vi "Code 0.0.5.vi"(8 "error in (no error)":errorcluster, 9 "Drv":u8(ring) items=["Drv 1", "Drv 2"], 10 "Port":u16=8030) -> (0 "error out":errorcluster)   [LabVIEW 2017]
panel:
  out "DataOut1":string
  out "DataOut2":string
  out "2":i32[][](array[numeric])
  out "1":i32[](array[numeric])
  in  "StopS.M. 2":bool
  in  "StopS.M.":bool
  in  "CatchNetworkFlag":bool
  in  "stop Listen":bool
  in  "status":bool
  out "conn ID":refnum<k5>
  out "Error List":string
  in  "Next Button":bool
  in  "File Path Control":path
  out "Status":bool
  out "CheckSum":bool[][](array[boolean])
  out "CheckSum DataB":u16 format="%.0x"
  out "CheckSum Data":u16 format="%.0x"
  out "Writting Data":bool
  out "Send Header":bool
  out "sumHeader":u16 format="%.0x"
  # "Ver 0.0.7"
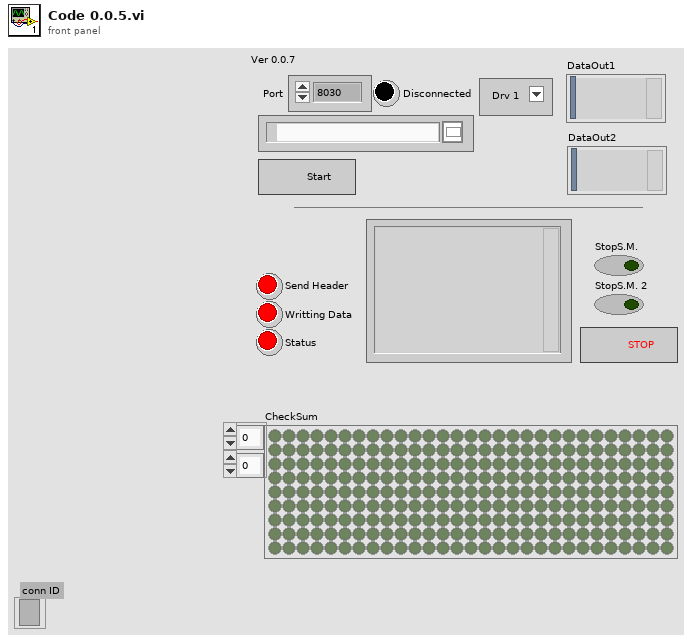
[diagram p1: front panel]
types:
  T1 = enum16{"open", "replace", "create", "open or create", "replace or create", "replace or create with confirmation"}
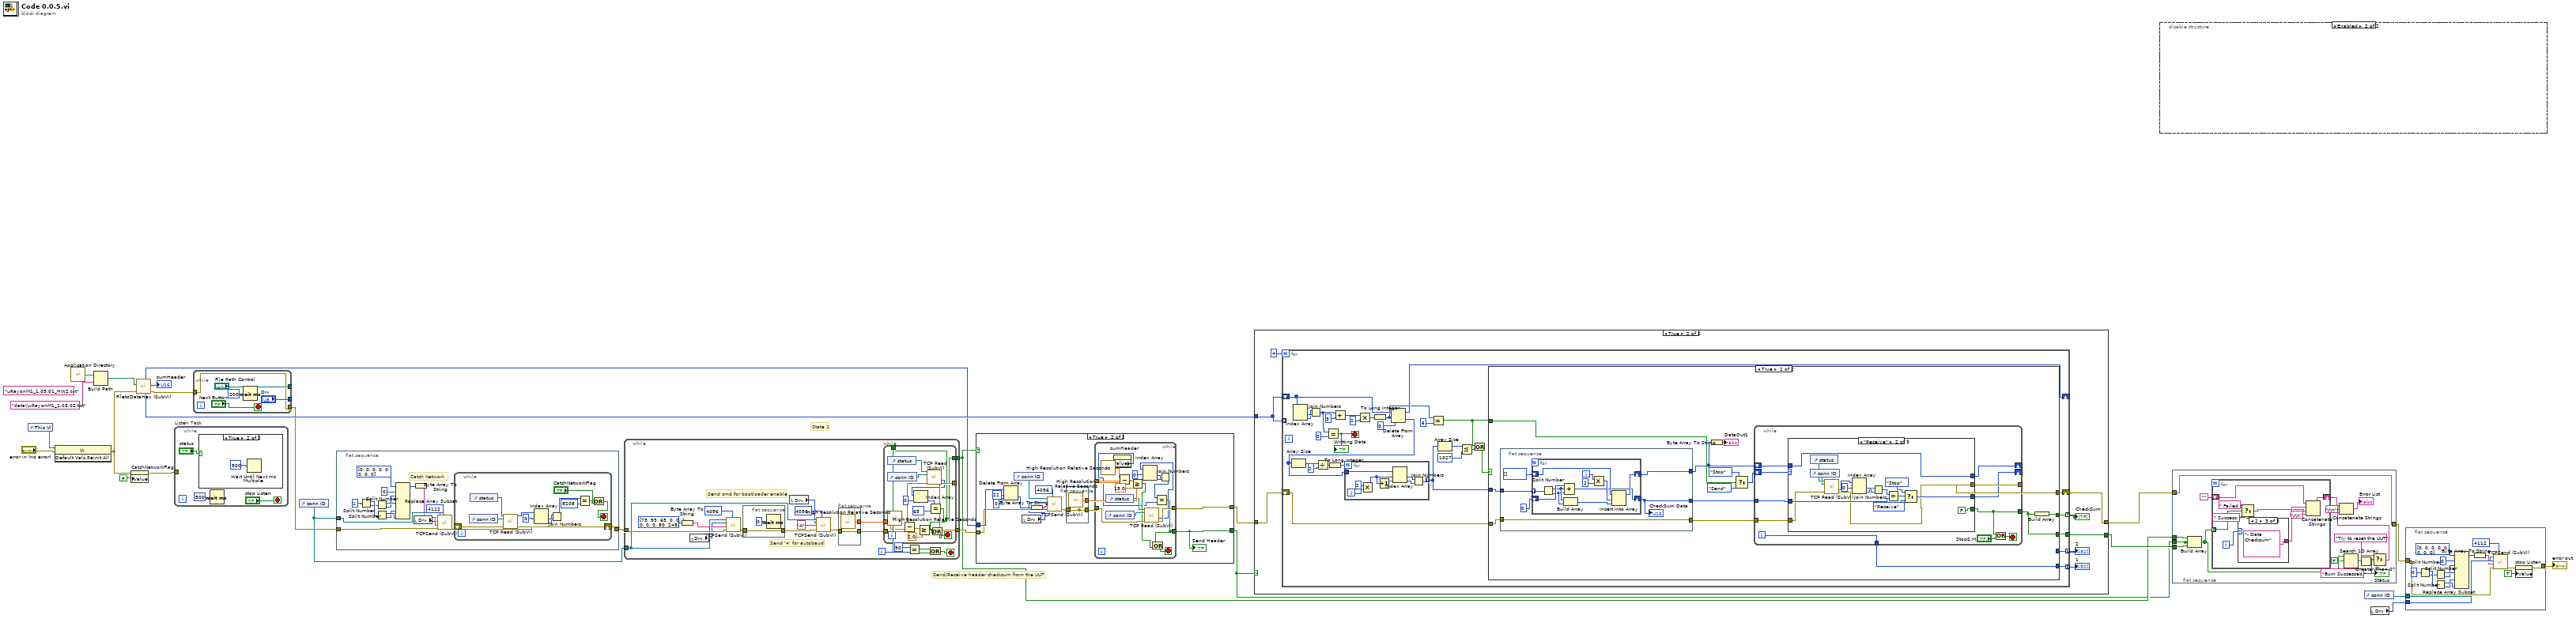
[diagram p0: block diagram]
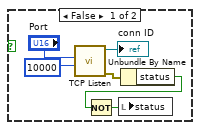
[diagram p2: hidden frame]
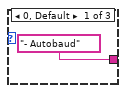
[diagram p3: hidden frame]
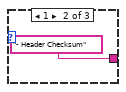
[diagram p4: hidden frame]
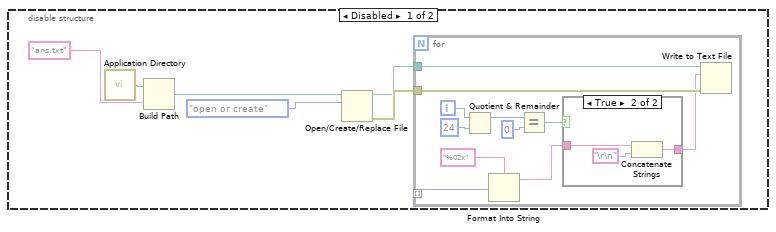
[diagram p5: hidden frame]
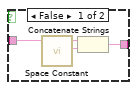
[diagram p6: hidden frame]
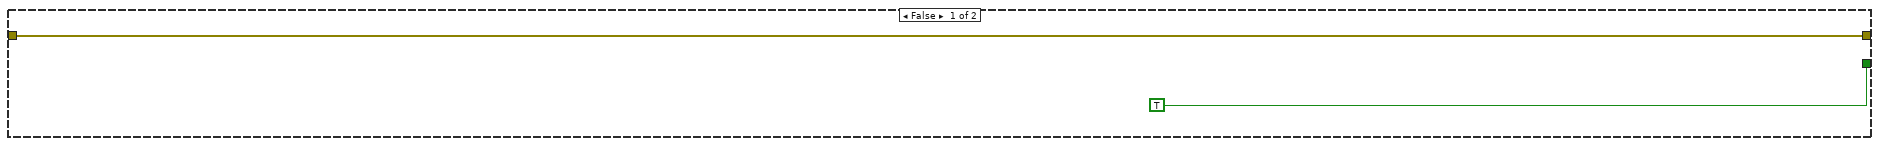
[diagram p7: hidden frame]
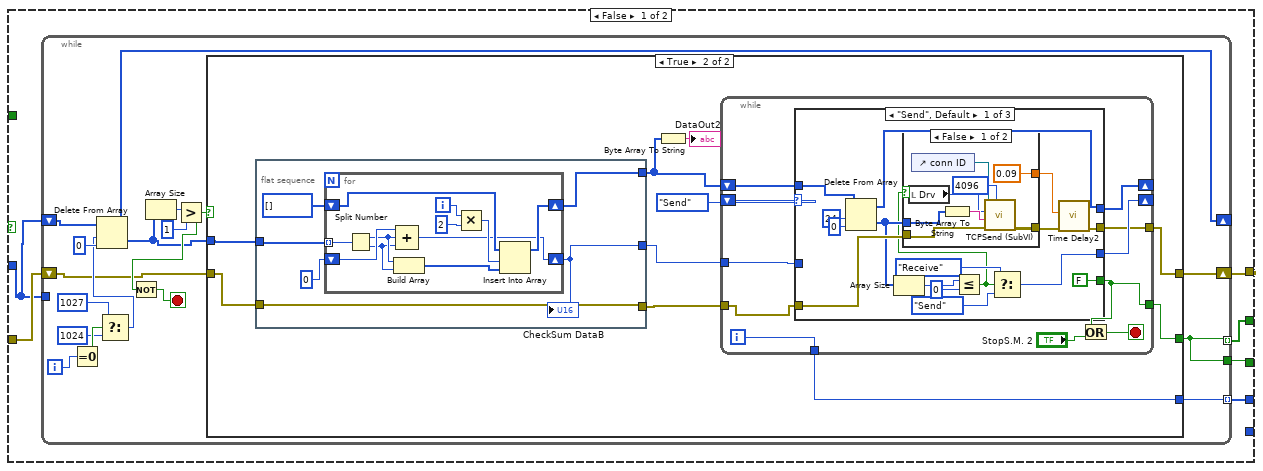
[diagram p8: hidden frame]
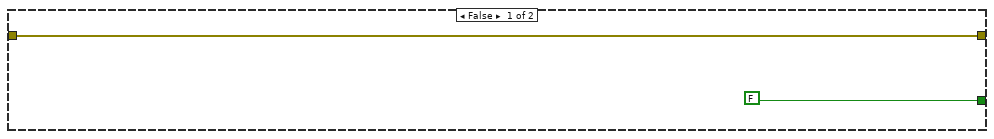
[diagram p9: hidden frame]
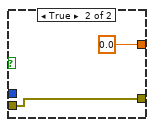
[diagram p10: hidden frame]
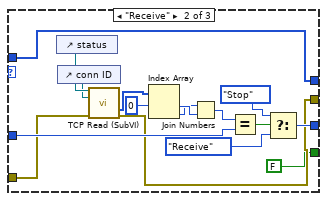
[diagram p11: hidden frame]
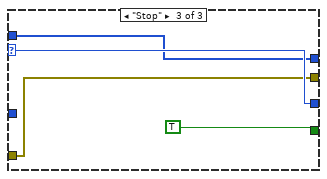
[diagram p12: hidden frame]
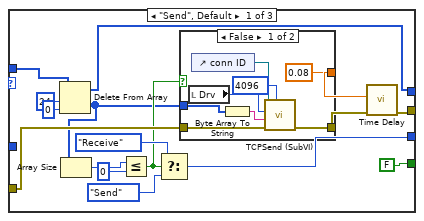
[diagram p13: hidden frame]
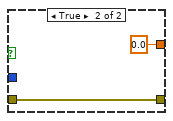
[diagram p14: hidden frame]
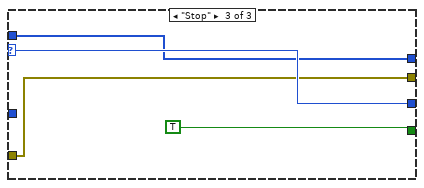
[diagram p15: hidden frame]
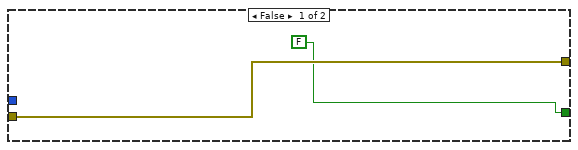
[diagram p16: hidden frame]
diagram:
  (unwired) "uRayonM1_1.05.01_HW2.txt" ("name or relative path")
  # "State 1"
  # "Send/Receive header checksum from the UUT"
  n1 = control-ref of="This VI"() -> (w24:refnum<vi>)
  n2 = invoke class="VI" method="Default Vals.Reinit All"(reference=w24, error in="error in (no error)") -> (error out=w4:errorcluster)  [unwired: 1 in, 2 out]
  n3 = call <vilib>:"Application Directory.vi"() -> ("Application Directory"=w8:path)
  n4 = Build Path(base path=w8, name or relative path="data\\uRayonM1_1.03.02.txt") -> (appended path=w7:path)
  n5 = property on="CatchNetworkFlag" class="Bool (strict)"(error in=w4, "Value"=FALSE ("stop")) -> (error out=w17:errorcluster)  [unwired: 1 in, 1 out]
  n6 = call "FiletoDataHex (SubVI).vi"("error constant"=w4, "file path (use dialog)"=w7) -> ("error constant 2"=w6:errorcluster, "Array 2"=w25:u8[], "Array"=w20:u8[], "sumHeader"=→"sumHeader":u16)  [unwired: 3 in, 3 out]
  n7 = while "Listen Task" {
    tunnel: w17 -> [_]
    stop <- "stop Listen" stop-if-true
    n8 = case shown="True" "status" {
      frame False {
        n9 = call <vilib>:"TCP Listen.vi"("timeout ms (wait forever: -1)"=10000, "port"="Port") -> ("error out"=w32:errorcluster, "connection ID"=→"conn ID":refnum<k5>)  [unwired: 5 in, 3 out]
        n10 = Unbundle By Name(w32) -> ("status"=w29:bool)
        n11 = Not(x=w29) -> (.not. x?=w30:bool)
        n12 = local write "status"(w30) -> ()
      }
      frame True {
        n13 = Wait Until Next ms Multiple(millisecond multiple=u32 500) -> ()  [unwired: 1 out]
      }
    }
    n14 = Wait (ms)(milliseconds to wait=u32 500) -> ()  [unwired: 1 out]
  }
  n15 = while {
    tunnel: ["File Path Control"] -> _
    tunnel: w6 -> [w36]
    tunnel: ["Drv"] -> _
    tunnel: [w36] -> w11
    stop <- "Next Button" stop-if-true
    n16 = Wait (ms)(milliseconds to wait=u32 200) -> ()  [unwired: 1 out]
  }
  n17 = control-ref of="conn ID"() -> (w13:refnum<vi>)
  n18 = flat-sequence {
    tunnel: w11 -> [w56]
    tunnel: w13 -> [w55]
    tunnel: [w43] -> w22
    frame #0 {
      # "Catch Network"
      n19 = Split Number(x=u32 1) -> (hi(x)=w53:u16, lo(x)=w52:u16)
      n20 = Split Number(x=w52) -> (hi(x)=w47:u8, lo(x)=w46:u8)
      n21 = Split Number(x=w53) -> (hi(x)=w45:u8, lo(x)=w44:u8)
      n22 = Replace Array Subset(array=u8[] [0, 0, 0, 0, 0, 0, 0, 0] ("unsigned byte array"), new element #1=w46, index #1=0 ("index"), new element #2=w47, new element #3=w44, new element #4=w45) -> (w48:u8[])  [unwired: 3 in]
      n23 = Byte Array To String(unsigned byte array=w48) -> (string=w54:string)
      n24 = local read "Drv"() -> (w41:u8)
      n25 = call "TCPSend (SubVI).vi"("Opcode"=u32 4112, "error in"=w56, "string"=w54, "Drv"=w41, "RefNum in"=w55) -> ("error out"=w42:errorcluster)  [unwired: 6 in]
      n26 = while {
        shift-right: [w69] -> w43
        shift-left: w42 -> [w70]
        stop <- w64 stop-if-true
        n27 = control-ref of="conn ID"() -> (w62:refnum<vi>)
        n28 = control-ref of="status"() -> (w63:refnum<vi>)
        n29 = call "TCP Read (SubVI).vi"("Status in"=w63, "TCP in"=w62, "error in (no error)"=w70) -> ("Rx data tmp"=w61:u8[], "error out"=w69:errorcluster)  [unwired: 2 in, 9 out]
        n30 = Index Array(array=w61, index #1=0 ("index")) -> (element #1=w60:u8, element #2=w59:u8)  [unwired: 1 in]
        n31 = Join Numbers(hi=w59, lo=w60) -> ((hi.lo)=w68:u16)
        n32 = Equal?(x=w68, y=u16 8208) -> (x = y?=w66:bool)
        n33 = Or(x="CatchNetworkFlag", y=w66) -> (x .or. y?=w64:bool)
      }
    }
  }
  n34 = while {
    tunnel: w22 -> [w84]
    tunnel: [w81] -> w16
    tunnel: w13 -> [w91]
    tunnel: [w80] -> w5
    i -> [w88]
    stop <- w90 stop-if-true
    # "Send 'A' for autobaud"
    # "Send cmd for bootloader enable"
    n35 = Byte Array To String(unsigned byte array=u8[] [73, 93, 65, 0, 0, 1, 0, 0, 0, 80, 248] ("output array")) -> (string=w76:string)
    n36 = local read "Drv"() -> (w71:u8)
    n37 = call "TCPSend (SubVI).vi"("Opcode"=u32 4096, "error in"=w84, "string"=w76, "Drv"=w71, "RefNum in"=w91) -> ("error out"=w78:errorcluster)  [unwired: 6 in]
    n38 = flat-sequence {
      tunnel: w78 -> [w92]
      tunnel: [w92] -> w77
      frame #0 {
        n39 = Wait (ms)(milliseconds to wait=u32 0) -> ()  [unwired: 1 out]
      }
    }
    n40 = local read "Drv"() -> (w72:u8)
    n41 = call "TCPSend (SubVI).vi"("Opcode"=u32 4096, "error in"=w77, "string"="A" ("write buffer"), "Drv"=w72, "RefNum in"=w91) -> ("error out"=w82:errorcluster)  [unwired: 6 in]
    n42 = flat-sequence {
      tunnel: w82 -> [w95]
      tunnel: [w95] -> w86
      tunnel: [w94] -> w85
      frame #0 {
        n43 = call <vilib>:"High Resolution Relative Seconds.vi"() -> ("relative seconds"=w94:dbl)
      }
    }
    n44 = while {
      tunnel: w86 -> [w99]
      tunnel: w85 -> [w105]
      tunnel: [w98] -> w81
      tunnel: [w96] -> w83
      tunnel: [w96] -> w80
      stop <- w97 stop-if-true
      n45 = control-ref of="status"() -> (w109:refnum<vi>)
      n46 = control-ref of="conn ID"() -> (w110:refnum<vi>)
      n47 = call <vilib>:"High Resolution Relative Seconds.vi"() -> ("relative seconds"=w106:dbl)
      n48 = Subtract(x=w106, y=w105) -> (x-y=w104:dbl)
      n49 = Greater Or Equal?(x=w104, y=2.0) -> (x >= y?=w102:bool)
      n50 = call "TCP Read (SubVI).vi"("Status in"=w109, "TCP in"=w110, "error in (no error)"=w99) -> ("Drv Array"=w107:u8[], "error out"=w98:errorcluster)  [unwired: 2 in, 9 out]
      n51 = Index Array(array=w107, index=0) -> (element=w101:u8)
      n52 = Equal?(x=w101, y=u8 65) -> (x = y?=w96:bool)
      n53 = Or(x=w96, y=w102) -> (x .or. y?=w97:bool)
    }
    n54 = Equal?(x=90, y=w88) -> (x = y?=w89:bool)
    n55 = Compound Arithmetic op=OR(w89, w83) -> (w90:bool)
  }
  n56 = case shown="True" w5 {
    tunnel: w16 -> [w112 w124]
    tunnel: [w112 w126] -> w2
    tunnel: w20 -> [_ w125]
    tunnel: [FALSE w114] -> w1
    frame False {
    }
    frame True {
      n57 = Delete From Array(array=w125, length=22, index=0) -> (deleted portion=w120:u8[])  [unwired: 1 out]
      n58 = control-ref of="conn ID"() -> (w117:refnum<vi>)
      n59 = local read "Drv"() -> (w113:u8)
      n60 = Byte Array To String(unsigned byte array=w120) -> (string=w118:string)
      n61 = call "TCPSend (SubVI).vi"("Opcode"=u32 4096, "error in"=w124, "string"=w118, "Drv"=w113, "RefNum in"=w117) -> ("error out"=w123:errorcluster)  [unwired: 6 in]
      n62 = flat-sequence {
        tunnel: w123 -> [w127]
        tunnel: [w127] -> _
        tunnel: [w128] -> w115
        tunnel: [w127] -> w116
        frame #0 {
          n63 = call <vilib>:"High Resolution Relative Seconds.vi"() -> ("relative seconds"=w128:dbl)
        }
      }
      n64 = while {
        tunnel: w116 -> [w139]
        tunnel: [w138] -> w126
        tunnel: w115 -> [w144]
        tunnel: [w129] -> w114
        stop <- w135 stop-if-true
        n65 = call <vilib>:"High Resolution Relative Seconds.vi"() -> ("relative seconds"=w145:dbl)
        n66 = control-ref of="status"() -> (w141:refnum<vi>)
        n67 = control-ref of="conn ID"() -> (w140:refnum<vi>)
        n68 = property on="sumHeader" class="DigNum (strict)"() -> ("Value"=w130:u16)  [unwired: 2 in, 2 out]
        n69 = Subtract(x=w145, y=w144) -> (x-y=w143:dbl)
        n70 = Greater Or Equal?(x=w143, y=15.0) -> (x >= y?=w134:bool)
        n71 = call "TCP Read (SubVI).vi"("Status in"=w141, "TCP in"=w140, "error in (no error)"=w139) -> ("Drv Array"=w136:u8[], "error out"=w138:errorcluster)  [unwired: 2 in, 9 out]
        n72 = Index Array(array=w136, index #1=0 ("index")) -> (element #1=w132:u8, element #2=w133:u8)  [unwired: 1 in]
        n73 = Join Numbers(hi=w133, lo=w132) -> ((hi.lo)=w131:u16)
        n74 = Equal?(x=w131, y=w130) -> (x = y?=w129:bool)
        n75 = Compound Arithmetic op=OR(w129, w134) -> (w135:bool)
      }
      "Send Header" <- w114
    }
  }
  n76 = case shown="True" w1 {
    tunnel: w2 -> [w147 w153]
    tunnel: [w147 w152] -> w19
    tunnel: w25 -> [_ w155]
    tunnel: [TRUE w151] -> w23
    frame False {
    }
    frame True {
      n77 = for {
        N: 4 -> [_]
        shift-right: [w176] -> _
        shift-left: w155 -> [w186]
        tunnel: w155 -> [_] mode=indexing
        tunnel: [w165] -> w154 mode=indexing
        shift-right: [w158] -> w152
        shift-left: w153 -> [w160]
        tunnel: [w159] -> w151
        tunnel: [w157] -> w149 mode=indexing
        tunnel: [w156] -> w148 mode=indexing
        stop <- w179 stop-if-true
        n78 = Index Array(array=w186) -> (element #1=w185:u8, element #2=w184:u8)  [unwired: 2 in]
        n79 = Join Numbers(hi=w184, lo=w185) -> ((hi.lo)=w162:u16)
        n80 = Equal?(x=w162, y=u16 0) -> (x = y?=w179:bool)
        "Writting Data" <- w179
        n81 = Add(x=w162, y=u32 3) -> (x+y=w182:u32)
        n82 = Multiply(x=w182, y=u32 2) -> (x*y=w180:u32)
        n83 = To Long Integer(number=w180) -> (32bit integer=w163:i32)
        n84 = Delete From Array(array=w186, length=w163, index=0) -> (deleted portion=w164:u8[], array with subset deleted=w176:u8[])
        n85 = Array Size(array=w164) -> (size(s)=w173:i32)
        n86 = Divide(x=w173, y=2) -> (x/y=w175:dbl)
        n87 = To Long Integer(number=w175) -> (32bit integer=w172:i32)
        n88 = for {
          N: w172 -> [_]
          tunnel: w164 -> [w388]
          tunnel: [w384] -> w169 mode=indexing
          i -> [w387]
          n89 = Multiply(x=2, y=w387) -> (x*y=w390:i32)
          n90 = Increment(x=w390) -> (x+1=w391:i32)
          n91 = Index Array(array=w388, index #1=w390, index #2=w391) -> (element #1=w386:u8, element #2=w385:u8)
          n92 = Join Numbers(hi=w386, lo=w385) -> ((hi.lo)=w384:u16)
        }
        n93 = Equal?(x=w163, y=6) -> (x = y?=w161:bool)
        n94 = Array Size(array=w169) -> (size(s)=w171:i32)
        n95 = Less Or Equal?(x=w171, y=1027) -> (x <= y?=w167:bool)
        n96 = Or(x=w161, y=w167) -> (x .or. y?=w166:bool)
        n97 = case shown="True" w166 {
          tunnel: w160 -> [w191 w307]
          tunnel: [w192 w304] -> w158
          tunnel: w169 -> [w189 w309]
          tunnel: [w190 w308] -> w165
          tunnel: w161 -> [_ w301]
          tunnel: [w188 w299] -> w159
          tunnel: [_ w298] -> w157
          tunnel: [w187 _] -> w156
          frame False {
            n98 = while {
              tunnel: w189 -> [_]
              tunnel: [w195] -> w190 mode=indexing
              shift-right: [w209] -> w192
              shift-left: w191 -> [w196]
              shift-right: [w202] -> _
              shift-left: w189 -> [w208]
              tunnel: [w195] -> w188
              tunnel: [w194] -> w187 mode=indexing
              i -> [w201]
              stop <- w203 stop-if-true
              n99 = Equal To 0?(x=w201) -> (x = 0?=w200:bool)
              n100 = Select(t=1027 ("length"), s=w200, f=1024 ("length")) -> (s? t:f=w197:i32)
              n101 = Delete From Array(array=w208, length=w197, index=0) -> (deleted portion=w193:u16[], array with subset deleted=w202:u16[])
              n102 = Array Size(array=w193) -> (size(s)=w206:i32)
              n103 = Greater?(x=w206, y=1) -> (0:w204:bool)
              n104 = Not(x=w204) -> (.not. x?=w203:bool)
              n105 = case shown="True" w204 {
                tunnel: [w211 w218] -> w209
                tunnel: w196 -> [w211 w220]
                tunnel: [FALSE w216] -> w195
                tunnel: w193 -> [_ w221]
                tunnel: [_ w214] -> w194
                frame False {
                }
                frame True {
                  n106 = flat-sequence {
                    tunnel: w220 -> [w280]
                    tunnel: [w282] -> w213
                    tunnel: [w279] -> w217
                    tunnel: w221 -> [w281]
                    tunnel: [w280] -> w215
                    frame #0 {
                      n107 = for {
                        tunnel: w281 -> [w295] mode=indexing
                        shift-right: [w290] -> w282
                        shift-left: u8[] [] -> [w289]
                        shift-right: [w287] -> w279
                        shift-left: u16 0 -> [w288]
                        i -> [w294]
                        n108 = Split Number(x=w295) -> (hi(x)=w286:u8, lo(x)=w285:u8)
                        n109 = Build Array(w286, w285) -> (w292:u8[])
                        n110 = Compound Arithmetic op=ADD(w288, w286, w285) -> (w287:u16)
                        n111 = Multiply(x=w294, y=2) -> (x*y=w291:i32)
                        n112 = Insert Into Array(array=w289, index=w291, new element=w292) -> (w290:u8[])
                      }
                      "CheckSum DataB" <- w279
                    }
                  }
                  n113 = Byte Array To String(unsigned byte array=w213) -> (string=→"DataOut2":string)
                  n114 = while {
                    shift-right: [w230] -> _
                    shift-left: enum16{"Stop", "Receive", "Send"}."Send" -> [w232]
                    shift-right: [w228] -> _
                    shift-left: w213 -> [w231]
                    tunnel: w215 -> [w223]
                    tunnel: w217 -> [w229]
                    tunnel: [w222] -> w216
                    tunnel: [w227] -> w218
                    tunnel: [w224] -> w214
                    i -> [w224]
                    stop <- w226 stop-if-true
                    n115 = case shown="\"Send\", Default" w232 {
                      selector: w232 -> [_ _ w278]
                      tunnel: w231 -> [w246 w263 w276]
                      tunnel: [w243 w265 w278] -> w230
                      tunnel: w223 -> [w242 w261 w275]
                      tunnel: w229 -> [_ w267 _]
                      tunnel: [FALSE FALSE TRUE] -> w222
                      tunnel: [w238 w263 w276] -> w228
                      tunnel: [w236 w262 w275] -> w227
                      frame "Send", Default {
                        n116 = Delete From Array(array=w246, length=24, index=0) -> (deleted portion=w235:u8[], array with subset deleted=w238:u8[])
                        n117 = Array Size(array=w235) -> (size(s)=w244:i32)
                        n118 = Less Or Equal?(x=w244, y=0) -> (x <= y?=w234:bool)
                        n119 = case shown="False" w234 {
                          tunnel: w235 -> [w252 _]
                          tunnel: w242 -> [w251 w258]
                          tunnel: [w250 w258] -> w237
                          tunnel: [0.09 ("Delay Time (s)") 0.0 ("Delay Time (s)")] -> w233
                          frame False {
                            n120 = local read "Drv"() -> (w253:u8)
                            n121 = control-ref of="conn ID"() -> (w254:refnum<vi>)
                            n122 = Byte Array To String(unsigned byte array=w252) -> (string=w255:string)
                            n123 = call "TCPSend (SubVI).vi"("Opcode"=u32 4096, "error in"=w251, "string"=w255, "Drv"=w253, "RefNum in"=w254) -> ("error out"=w250:errorcluster)  [unwired: 6 in]
                          }
                          frame True {
                          }
                        }
                        n124 = Select(t=enum16{"Stop", "Receive", "Send"}."Receive", s=w234, f=enum16{"Stop", "Receive", "Send"}."Send") -> (s? t:f=w243:enum16{"Stop", "Receive", "Send"})
                        n125 = call "Time Delay2"("error in (no error)"=w237, "Delay Time (s)"=w233) -> ("error out"=w236:errorcluster)  [unwired: 9 in]
                      }
                      frame "Receive" {
                        n126 = control-ref of="status"() -> (w274:refnum<vi>)
                        n127 = control-ref of="conn ID"() -> (w273:refnum<vi>)
                        n128 = call "TCP Read (SubVI).vi"("Status in"=w274, "TCP in"=w273, "error in (no error)"=w261) -> ("Drv Array"=w269:u8[], "error out"=w262:errorcluster)  [unwired: 2 in, 9 out]
                        n129 = Index Array(array=w269, index #1=0 ("index")) -> (element #1=w272:u8, element #2=w271:u8)  [unwired: 1 in]
                        n130 = Join Numbers(hi=w271, lo=w272) -> ((hi.lo)=w268:u16)
                        n131 = Equal?(x=w268, y=w267) -> (x = y?=w260:bool)
                        n132 = Select(t=enum16{"Stop", "Receive", "Send"}."Stop", s=w260, f=enum16{"Stop", "Receive", "Send"}."Receive") -> (s? t:f=w265:enum16{"Stop", "Receive", "Send"})
                      }
                      frame "Stop" {
                      }
                    }
                    n133 = Or(x=w222, y="StopS.M. 2") -> (x .or. y?=w226:bool)
                  }
                }
              }
            }
          }
          frame True {
            n134 = flat-sequence {
              tunnel: w307 -> [w368]
              tunnel: [w370] -> w296
              tunnel: w309 -> [w369]
              tunnel: [w368] -> w306
              tunnel: [w367] -> w305
              frame #0 {
                n135 = for {
                  tunnel: w369 -> [w383] mode=indexing
                  shift-right: [w378] -> w370
                  shift-left: u8[] [] -> [w377]
                  shift-right: [w375] -> w367
                  shift-left: u16 0 -> [w376]
                  i -> [w382]
                  n136 = Split Number(x=w383) -> (hi(x)=w374:u8, lo(x)=w373:u8)
                  n137 = Build Array(w374, w373) -> (w380:u8[])
                  n138 = Compound Arithmetic op=ADD(w376, w374, w373) -> (w375:u16)
                  n139 = Multiply(x=w382, y=2) -> (x*y=w379:i32)
                  n140 = Insert Into Array(array=w377, index=w379, new element=w380) -> (w378:u8[])
                }
                "CheckSum Data" <- w367
              }
            }
            n141 = Byte Array To String(unsigned byte array=w296) -> (string=→"DataOut1":string)
            n142 = Select(t=enum16{"Stop", "Receive", "Send"}."Stop", s=w301, f=enum16{"Stop", "Receive", "Send"}."Send") -> (s? t:f=w302:enum16{"Stop", "Receive", "Send"})
            n143 = while {
              shift-right: [w318] -> _
              shift-left: w302 -> [w320]
              shift-right: [w315] -> _
              shift-left: w296 -> [w319]
              tunnel: w306 -> [w317]
              tunnel: w305 -> [w316]
              tunnel: [w314] -> w299
              tunnel: [w313] -> w304
              tunnel: [w310] -> w298
              i -> [w310]
              stop <- w312 stop-if-true
              n144 = case shown="\"Receive\"" w320 {
                selector: w320 -> [_ _ w366]
                tunnel: w319 -> [w334 w350 w364]
                tunnel: [w331 w352 w366] -> w318
                tunnel: w317 -> [w330 w348 w363]
                tunnel: w316 -> [_ w355 _]
                tunnel: [FALSE FALSE TRUE] -> w314
                tunnel: [w326 w350 w364] -> w315
                tunnel: [w324 w349 w363] -> w313
                frame "Send", Default {
                  n145 = Delete From Array(array=w334, length=24, index=0) -> (deleted portion=w322:u8[], array with subset deleted=w326:u8[])
                  n146 = Array Size(array=w322) -> (size(s)=w332:i32)
                  n147 = Less Or Equal?(x=w332, y=0) -> (x <= y?=w323:bool)
                  n148 = Select(t=enum16{"Stop", "Receive", "Send"}."Receive", s=w323, f=enum16{"Stop", "Receive", "Send"}."Send") -> (s? t:f=w331:enum16{"Stop", "Receive", "Send"})
                  n149 = case shown="False" w323 {
                    tunnel: w322 -> [w340 _]
                    tunnel: w330 -> [w339 w346]
                    tunnel: [w338 w346] -> w325
                    tunnel: [0.08 ("Delay Time (s)") 0.0 ("Delay Time (s)")] -> w321
                    frame False {
                      n150 = local read "Drv"() -> (w341:u8)
                      n151 = control-ref of="conn ID"() -> (w342:refnum<vi>)
                      n152 = Byte Array To String(unsigned byte array=w340) -> (string=w343:string)
                      n153 = call "TCPSend (SubVI).vi"("Opcode"=u32 4096, "error in"=w339, "string"=w343, "Drv"=w341, "RefNum in"=w342) -> ("error out"=w338:errorcluster)  [unwired: 6 in]
                    }
                    frame True {
                    }
                  }
                  n154 = call "Time Delay"("error in (no error)"=w325, "Delay Time (s)"=w321) -> ("error out"=w324:errorcluster)  [unwired: 9 in]
                }
                frame "Receive" {
                  n155 = control-ref of="status"() -> (w362:refnum<vi>)
                  n156 = control-ref of="conn ID"() -> (w361:refnum<vi>)
                  n157 = call "TCP Read (SubVI).vi"("Status in"=w362, "TCP in"=w361, "error in (no error)"=w348) -> ("Drv Array"=w357:u8[], "error out"=w349:errorcluster)  [unwired: 2 in, 9 out]
                  n158 = Index Array(array=w357, index #1=0 ("index")) -> (element #1=w360:u8, element #2=w359:u8)  [unwired: 1 in]
                  n159 = Join Numbers(hi=w359, lo=w360) -> ((hi.lo)=w356:u16)
                  n160 = Equal?(x=w356, y=w355) -> (x = y?=w354:bool)
                  n161 = Select(t=enum16{"Stop", "Receive", "Send"}."Stop", s=w354, f=enum16{"Stop", "Receive", "Send"}."Receive") -> (s? t:f=w352:enum16{"Stop", "Receive", "Send"})
                }
                frame "Stop" {
                }
              }
              n162 = Or(x=w314, y="StopS.M.") -> (x .or. y?=w312:bool)
            }
            n163 = Build Array(w299) -> (w308:bool[])
          }
        }
      }
      "CheckSum" <- w154
      "1" <- w149
      "2" <- w148
    }
  }
  n164 = disable-structure shown="Enabled" {
    frame Disabled {
      n165 = call <vilib>:"Application Directory.vi"() -> ("Application Directory"=w396:path)
      n166 = Build Path(base path=w396, name or relative path="ans.txt") -> (appended path=w395:path)
      n167 = Open/Create/Replace File(file path (use dialog)=w395, operation (0:open)=T1."open or create") -> (refnum out=w392:refnum<file>, error out=w393:errorcluster)  [unwired: 4 in, 1 out]
      n168 = for {
        tunnel: _ -> [w408] mode=indexing
        tunnel: w393 -> [w406]
        tunnel: w392 -> [w405]
        i -> [w401]
        n169 = Quotient & Remainder(x=w401, y=24 ("x")) -> (x-y*floor(x/y)=w399:i32)  [unwired: 1 out]
        n170 = Format Into String(format string="%02x", w408) -> (resulting string=w404:string)  [unwired: 2 in, 1 out]
        n171 = Equal?(x=w399, y=0) -> (x = y?=w402:bool)
        n172 = case shown="True" w402 {
          tunnel: w404 -> [w411 w414]
          tunnel: [w410 w413] -> w403
          frame False {
            n173 = call <vilib>:"Space Constant.vi"() -> ("String"=w409:string)
            n174 = Concatenate Strings(w411, w409) -> (w410:string)
          }
          frame True {
            n175 = Concatenate Strings(w414, "\r\n") -> (w413:string)
          }
        }
        n176 = Write to Text File(file (use dialog)=w405, text=w403, error in=w406) -> ()  [unwired: 1 in, 3 out]
      }
    }
    frame Enabled {
    }
  }
  n177 = flat-sequence {
    tunnel: w19 -> [w429]
    tunnel: [w429] -> w15
    tunnel: w5 -> [w428]
    tunnel: [w416] -> _
    tunnel: w23 -> [w427]
    tunnel: w1 -> [w416]
    frame #0 {
      n178 = Build Array(w428, w416, w427) -> (w422:bool[])
      n179 = for {
        tunnel: w422 -> [w438] mode=indexing
        shift-right: [w436] -> w425
        shift-left: "" -> [w437]
        i -> [w434]
        n180 = case shown="2" w434 {
          tunnel: ["- Autobaud" "- Header Checksum" "- Data Checksum"] -> w431
          frame 0, Default {
          }
          frame 1 {
          }
          frame 2 {
          }
        }
        n181 = Select(t=" Failed !", s=w438, f=" Success !") -> (s? t:f=w430:string)
        n182 = Concatenate Strings(w437, w431, w430, "\r\n") -> (w436:string)
      }
      n183 = Search 1D Array(1D array=w422, element=TRUE) -> (index of element=w420:i32)  [unwired: 1 in]
      n184 = Greater Than 0?(x=w420) -> (x > 0?=w415:bool)
      "Status" <- w415
      n185 = Select(t="Try to reset the UUT" ("string"), s=w415, f="Burn Successed.") -> (s? t:f=w418:string)
      n186 = Concatenate Strings(w425, "\r\n", w418) -> (→"Error List":string)
    }
  }
  n187 = control-ref of="conn ID"() -> (w12:refnum<vi>)
  n188 = local read "Drv"() -> (w3:u8)
  n189 = flat-sequence {
    tunnel: w15 -> [w459]
    tunnel: w3 -> [w458]
    tunnel: w12 -> [w457]
    tunnel: [w442] -> w14
    frame #0 {
      n190 = Split Number(x=u32 0) -> (hi(x)=w455:u16, lo(x)=w454:u16)
      n191 = Split Number(x=w454) -> (hi(x)=w449:u8, lo(x)=w448:u8)
      n192 = Split Number(x=w455) -> (hi(x)=w447:u8, lo(x)=w446:u8)
      n193 = Replace Array Subset(array=u8[] [0, 0, 0, 0, 0, 0, 0, 0] ("unsigned byte array"), new element #1=w448, index #1=0 ("index"), new element #2=w449, new element #3=w446, new element #4=w447) -> (w450:u8[])  [unwired: 3 in]
      n194 = Byte Array To String(unsigned byte array=w450) -> (string=w444:string)
      n195 = call "TCPSend (SubVI).vi"("Opcode"=u32 4112, "error in"=w459, "string"=w444, "Drv"=w458, "RefNum in"=w457) -> ("error out"=w456:errorcluster)  [unwired: 6 in]
      n196 = property on="stop Listen" class="Bool (strict)"(error in=w456, "Value"=TRUE ("stop Listen")) -> (error out=w442:errorcluster)  [unwired: 1 in, 1 out]
    }
  }
  "error out" <- w14
